vi "DAC Run.vi"(8 "error in":errorcluster, 11 "DAC TC Temperature in":refnum<class "DAC TC Temp DeepU.lvclass">) -> (0 "error out":errorcluster, 3 "DAC TC Temperature out":refnum<class "DAC TC Temp DeepU.lvclass">)   [LabVIEW 2019, in "DAC.lvlib" / "DAC TC Temp DeepU.lvclass"]
uses:
  DAC TC Temp DeepU.lvclass
  C:/Users/krio/Documents/LV_Projects/test-stand/App/DAC/DAC.lvclass
  DAC.lvclass/DAC.ctl
  Results/Results Method.ctl
  Results/DeepU Results/DeepU Results.lvclass
  DAC TC Temp DeepU.lvclass/DAC TC Temp DeepU.ctl
  <vilib>/DAQmx/read.llb/DAQmx Read (Analog 1D Wfm NChan 1Samp).vi
  <vilib>/DAQmx/miscellaneous.llb/DAQmx Fill In Error Info.vi
  DAC.lvclass
  Results/Results.lvlib
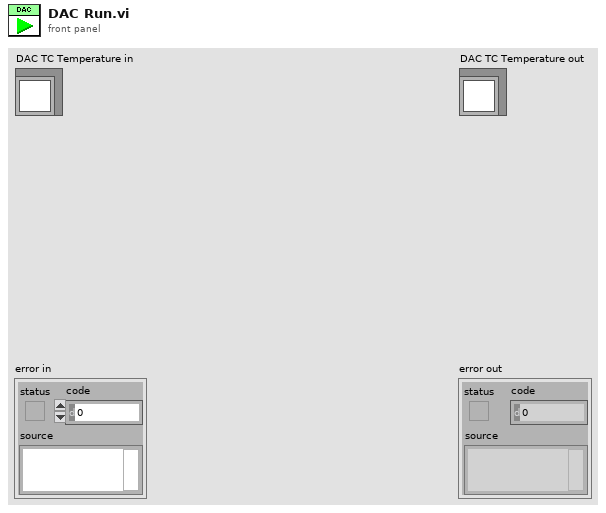
[diagram p1: front panel]
types:
  T1 = typedef "Results.lvlib/Results Method.ctl" = enum16{"Get", "Set"}
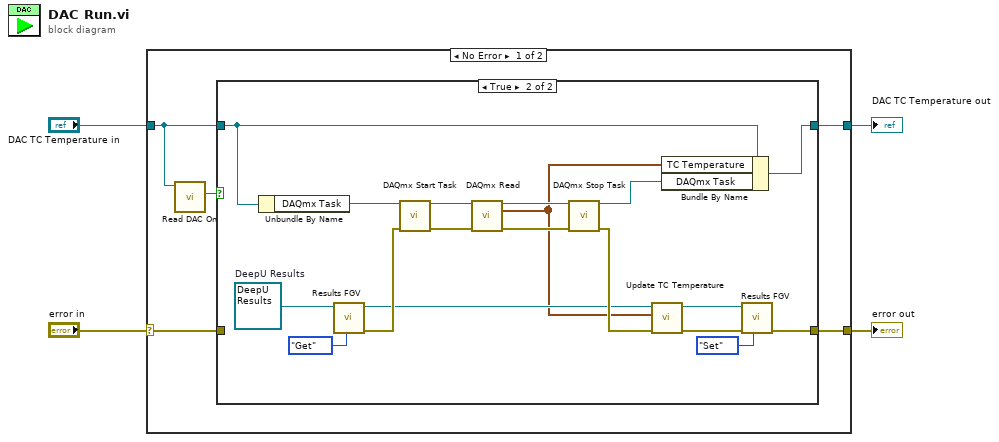
[diagram p0: block diagram]
diagram:
  n1 = case shown="No Error" "error in" {
    selector: "error in" -> [w7 w31]
    tunnel: [w6 w31] -> w2
    tunnel: [w8 w30] -> w1
    tunnel: "DAC TC Temperature in" -> [w5 w30]
    frame No Error {
      n2 = call "Read DAC On.vi"("DAC in"=w5) -> ("DAC On"=w9:bool)  [unwired: 8 in, 2 out]
      n3 = case shown="True" w9 {
        tunnel: w5 -> [w11 w24]
        tunnel: [w11 w23] -> w8
        tunnel: w7 -> [w10 _]
        tunnel: [w10 w18] -> w6
        frame False {
        }
        frame True {
          w21 = refnum<class "DeepU Results.lvclass"> refnum  # DeepU Results
          n4 = Unbundle By Name(w24) -> ("DAQmx Task"=w29:refnum<k21>)
          n5 = call-dynamic "Results FGV.vi"("Method"=Results_Method."Get", "DeepU Results in"=w21) -> ("error out"=w17:errorcluster, "DeepU Results out"=w14:refnum<class "DeepU Results.lvclass">)  [unwired: 8 in]
          n6 = call <vilib>:"DAQmx Start Task.vi"("task/channels in"=w29, "error in"=w17) -> ("task out"=w28:refnum<k21>, "error out"=w26:errorcluster)  [unwired: 12 in]
          n7 = call-poly <vilib>:"DAQmx Read.vi"("task/channels in"=w28, "error in"=w26) -> ("task out"=w27:refnum<k21>, "data"=w12:waveform(dbl)[], "error out"=w25:errorcluster)  [unwired: 11 in]
          n8 = call <vilib>:"DAQmx Stop Task.vi"("task/channels in"=w27, "error in"=w25) -> ("task out"=w22:refnum<k21>, "error out"=w15:errorcluster)  [unwired: 12 in]
          n9 = call "Update TC Temperature.vi"("error in"=w15, "TC Temperature"=w12, "DeepU Results in"=w14) -> ("error out"=w16:errorcluster, "DeepU Results out"=w13:refnum<class "DeepU Results.lvclass">)  [unwired: 7 in]
          n10 = Bundle By Name(cluster=w24, "TC Temperature"=w12, "DAQmx Task"=w22) -> (w23:refnum<class "DAC TC Temp DeepU.lvclass">)
          n11 = call-dynamic "Results FGV.vi"("Method"=Results_Method."Set", "error in"=w16, "DeepU Results in"=w13) -> ("error out"=w18:errorcluster)  [unwired: 7 in, 1 out]
        }
      }
    }
    frame Error {
    }
  }
  "error out" <- w2
  "DAC TC Temperature out" <- w1
